vi "poly_wait_for_value_change_single.vi"(6 "timeout (never)":i32=-1, 8 "error in":errorcluster, 9 "stop ref":refnum<vi>, 10 "control ref":refnum<vi>) -> (0 "error out":errorcluster, 2 "timed out?":bool)   [LabVIEW 2015]
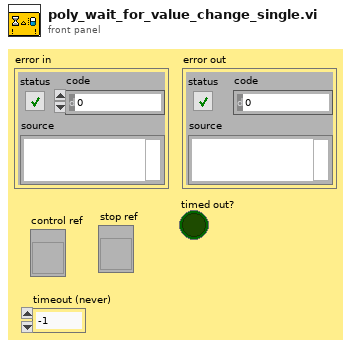
[diagram p1: front panel]
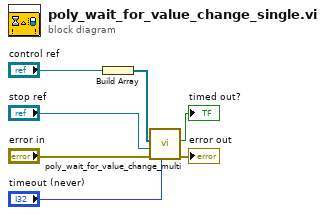
[diagram p0: block diagram]
diagram:
  n1 = Build Array("control ref") -> (w6:refnum<vi>[])
  n2 = call "poly_wait_for_value_change_multi.vi"("timeout (never)"="timeout (never)", "error in"="error in", "stop ref"="stop ref", "control ref"=w6) -> ("error out"=→"error out":errorcluster, "timed out?"=→"timed out?":bool)  [unwired: 6 in]
